vi "Get Column Headers.vi"() -> (3 "Headers":string[](array[string]))   [LabVIEW 2019, in "STS_LTRV.lvlib"]
uses:
  STS_LTRV.lvlib
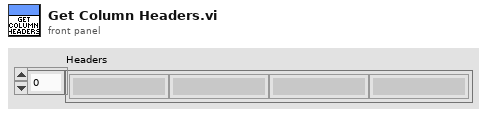
[diagram p1: front panel]
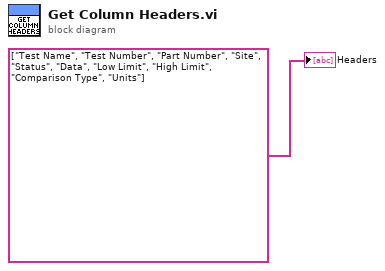
[diagram p0: block diagram]
diagram:
  "Headers" <- string[] ["Test Name", "Test Number", "Part Number", "Site", "Status", "Data", "Low Limit", "High Limit", "Comparison Type", "Units"] ("Headers")
